vi "Configure Trigger.vi"(8 "error in (no error)":errorcluster, 10 "Source":string, 11 "Camera in":refnum<class "Camera.lvclass">) -> (0 "error out":errorcluster, 3 "Camera":refnum<class "Camera.lvclass">)   [LabVIEW 2020, in "Camera.lvclass"]
uses:
  Camera.lvclass
  Camera.lvclass/Camera.ctl
  bin/gindustrialcam_32-1.dll
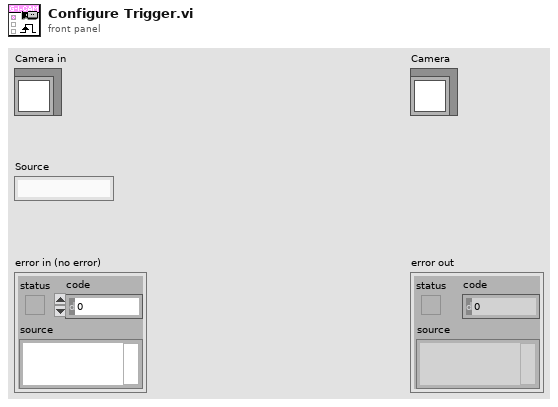
[diagram p1: front panel]
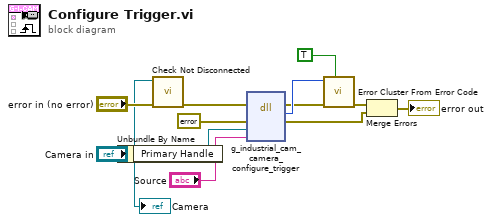
[diagram p0: block diagram]
diagram:
  n1 = Unbundle By Name("Camera in") -> ("Primary Handle"=w8:refnum<data-value>)
  n2 = call "Check Not Disconnected.vi"("error in (no error)"="error in (no error)", "Camera in"="Camera in") -> ("error out"=w7:errorcluster)  [unwired: 9 in]
  n3 = dll-call lib="C:/serenial/lib/g-industrial-camera/LabVIEW/g_industrial_cam/bin/gindustrialcam_*-1.*" fn="g_industrial_cam_camera_configure_trigger"(error in=w7, "err"=errorcluster {"status"=FALSE, "code"=0, "source"=""} ("error constant"), "edvr"=w8, "formats"="Source") -> (error out=w1:errorcluster, "Mg_Error"=w2:i32, "err"=w4:errorcluster)  [unwired: 4 in, 1 out]
  n4 = call <vilib>:"Error Cluster From Error Code.vi"("show call chain? (False)"=TRUE, "error in (no error)"=w1, "error code (0)"=w2) -> ("error out"=w3:errorcluster)  [unwired: 6 in]
  n5 = Merge Errors(w3, w4) -> (→"error out":errorcluster)
  "Camera" <- "Camera in"
